vi "read Array of Double.vi"(10 "index":i32, 11 "data table in":T1) -> (1 "value":dbl[](array[numeric]), 3 "data table out":T1)   [LabVIEW 2013, in "data bus values.lvlib"]
doc: "Reads a single value from the data table."
uses:
  data bus values.lvlib
  data table.ctl
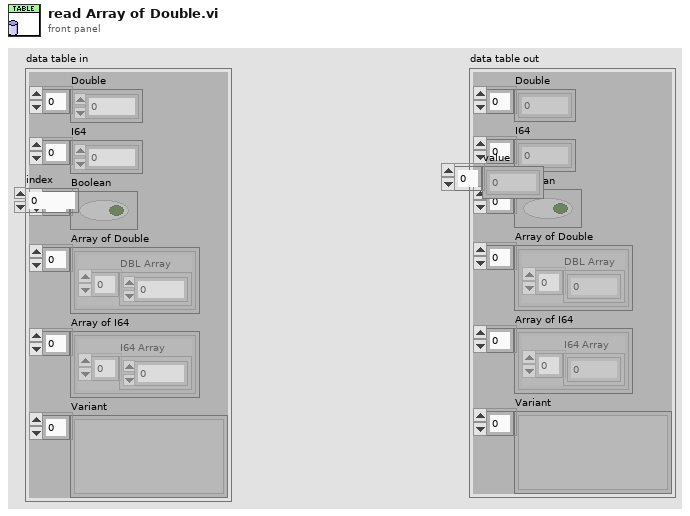
[diagram p1: front panel]
types:
  T1 = typedef "data bus values.lvlib/data table.ctl" = cluster{"Double":dbl[], "I64":i64[], "Boolean":bool[], "Array of Double":cluster{"DBL Array":dbl[]}[], "Array of I64":cluster{"I64 Array":i64[]}[], "Variant":variant[]}
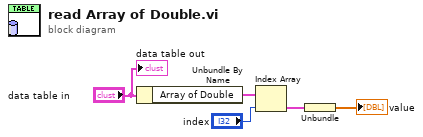
[diagram p0: block diagram]
diagram:
  n1 = Unbundle By Name("data table in") -> ("Array of Double"=w4:cluster{"DBL Array":dbl[]}[])
  n2 = Index Array(array=w4, index="index") -> (element=w2:cluster{"DBL Array":dbl[]})
  n3 = Unbundle(w2) -> ("DBL Array"=→"value":dbl[])
  "data table out" <- "data table in"
